vi "LabVIEW Data to Python String (Variant)-[no 2d array support].vi"(8 "error in (no error)":errorcluster, 10 "LabVIEW Data":variant) -> (0 "error out":errorcluster, 2 "Python String":string)   [LabVIEW 2020, in "jki_python_data_tools.lvlib"]
doc: "Writes a value associated with key in a specified section of the configuration data identified by refnum. If \"key\" input is not specified, the name of the variant object is used as the key.\n\nFor example a Boolean named \"Enable\" with a value of TRUE would correspond to the key-value pair:\n\nEnable=TRUE"
uses:
  jki_python_data_tools.lvlib
  LabVIEW Data to Python String/LabVIEW Data to Python String (I64).vi
  LabVIEW Data to Python String/LabVIEW Data to Python String (U64).vi
  LabVIEW Data to Python String/LabVIEW Data to Python String (Boolean).vi
  LabVIEW Data to Python String/LabVIEW Data to Python String (EXT).vi
  LabVIEW Data to Python String/LabVIEW Data to Python String (CXT).vi
  LabVIEW Data to Python String/LabVIEW Data to Python String (Path).vi
  LabVIEW Data to Python String/LabVIEW Data to Python String (String).vi
  LabVIEW Data to Python String/LabVIEW Data to Python String (I32).vi
  LabVIEW Data to Python String/LabVIEW Data to Python String (U32).vi
panel:
  # "Copyright © 2003-2009 JKI. All rights reserved.\n\nAuthor: Jim Kring [jim.kring@jameskring.com]\n\nThis library is provided \"AS IS\" ,WITHOUT WARRANTIES OR \nCONDITIONS OF ANY KIND, either express or implied.\n\nJames Kring, Inc. -- http://www.jameskring.com"
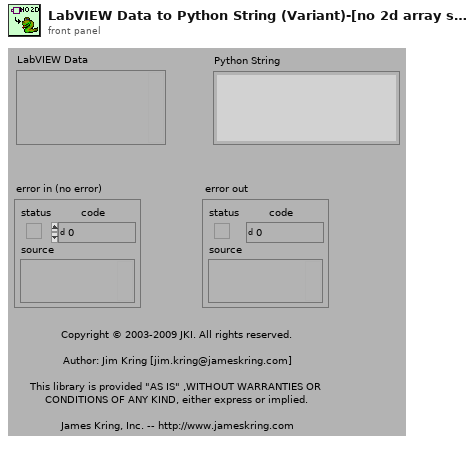
[diagram p1: front panel]
types:
  T1 = typedef "jki_python_data_tools.lvlib/Type Descriptor Enumeration__Py2LV.ctl" = enum8{"<Null>", "I8", "I16", "I32", "I64", "U8", "U16", "U32", "U64", "SGL", "DBL", "EXT", "CSG", "CDB", "CXT", "0x0F", "0x10", "0x11", "0x12", "0x13", "0x14", "Enum U8", "Enum U16", "Enum U32", "Enum U64", "SGL PQ", "DBL PQ", "EXT PQ", "CSG PQ", "CDB PQ", "CXT PQ", "0x1F", "0x20", "Boolean", "0x22", "0x23", "0x24", "0x25", "0x26", "0x27", "0x28", "0x29", "0x2A", "0x2B", "0x2C", "0x2D", "0x2E", "0x2F", "String", "0x31", "Path", "Pict", "0x34", "0x35", "0x36", "DAQ", "0x38", "0x39", "0x3A", "0x3B", "0x3C", "0x3D", "0x3E", "0x3F", "Array", "0x41", "0x42", "0x43", "0x44", "0x45", "0x46", "0x47", "0x48", "0x49", "0x4A", "0x4B", "0x4C", "0x4D", "0x4E", "0x4F", "Cluster", "0x51", "0x52", "Variant", "Waveform", "0x55", "0x56", "0x57", "0x58", "0x59", "0x5A", "0x5B", "0x5C", "0x5D", "0x5E", "0x5F", "0x60", "0x61", "0x62", "0x63", "0x64", "0x65", "0x66", "0x67", "0x68", "0x69", "0x6A", "0x6B", "0x6C", "0x6D", "0x6E", "0x6F", "Refnum"}
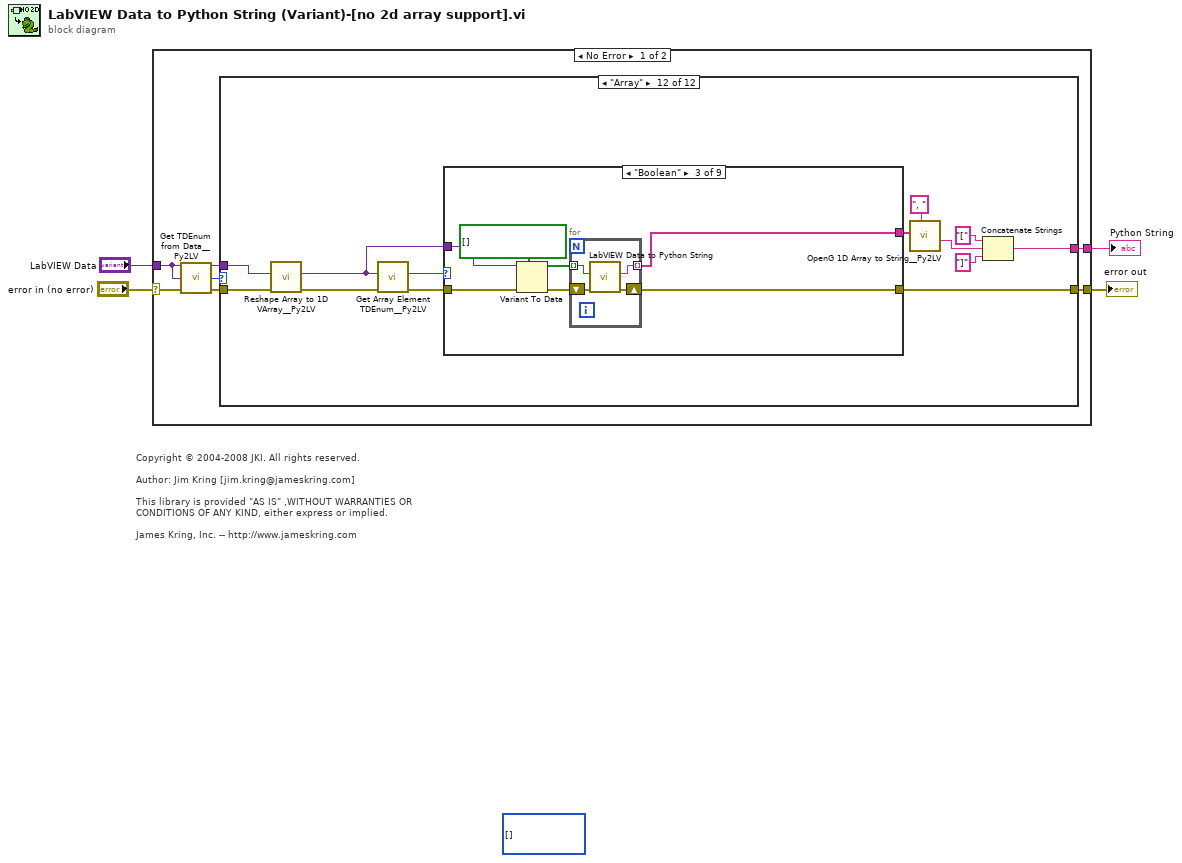
[diagram p0: block diagram]
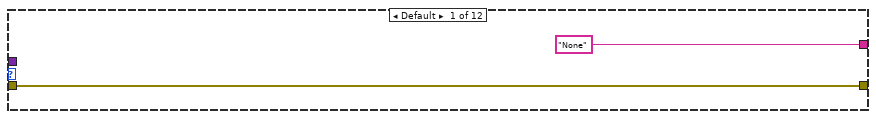
[diagram p2: hidden frame]
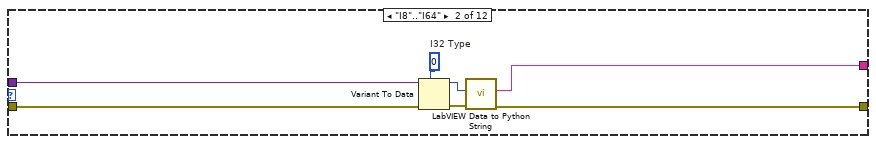
[diagram p3: hidden frame]
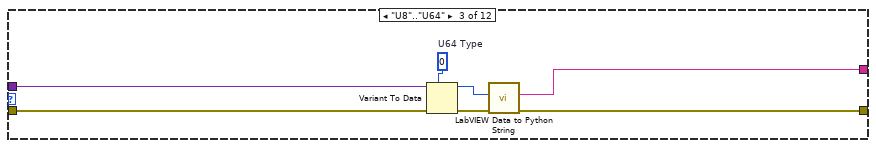
[diagram p4: hidden frame]
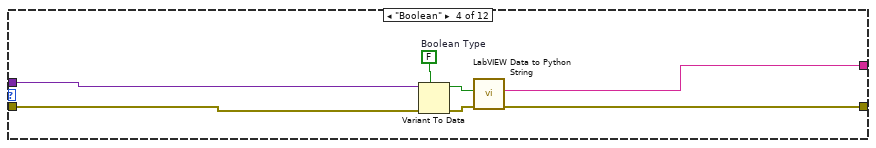
[diagram p5: hidden frame]
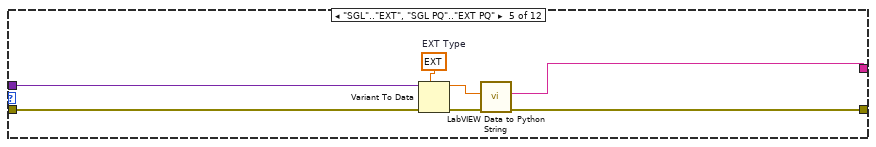
[diagram p6: hidden frame]
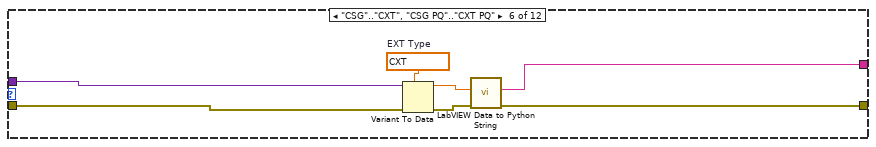
[diagram p7: hidden frame]
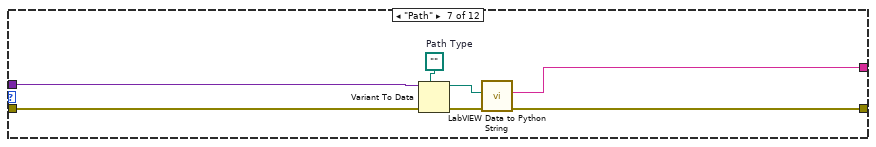
[diagram p8: hidden frame]
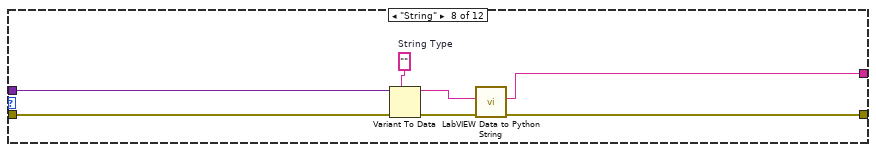
[diagram p9: hidden frame]
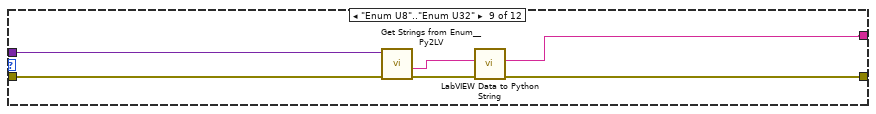
[diagram p10: hidden frame]
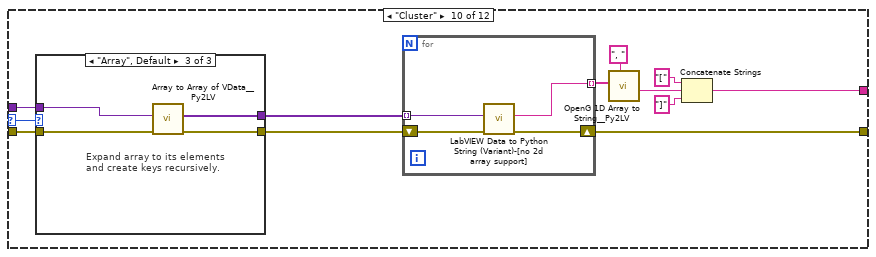
[diagram p11: hidden frame]
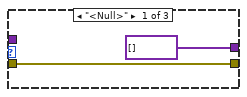
[diagram p12: hidden frame]
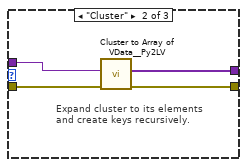
[diagram p13: hidden frame]
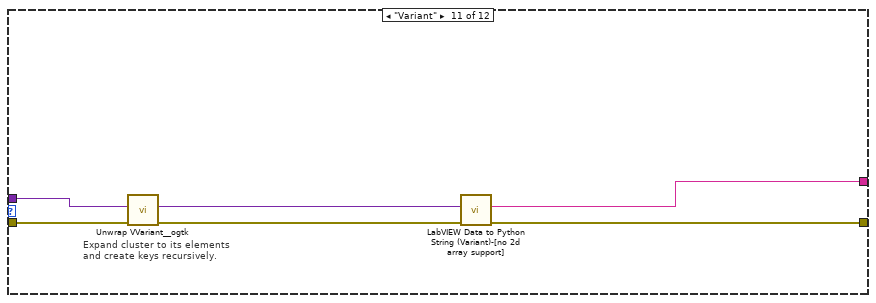
[diagram p14: hidden frame]
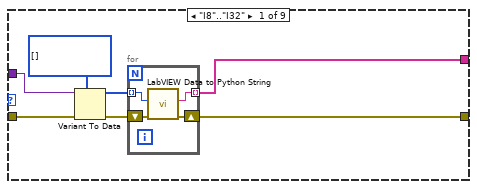
[diagram p15: hidden frame]
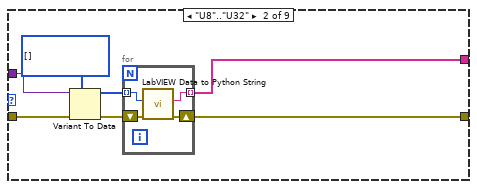
[diagram p16: hidden frame]
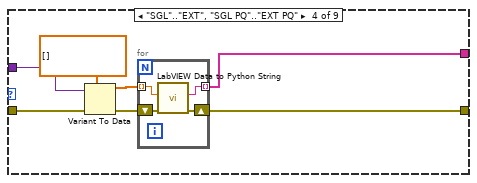
[diagram p17: hidden frame]
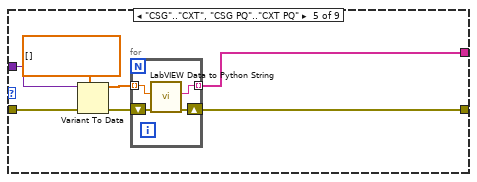
[diagram p18: hidden frame]
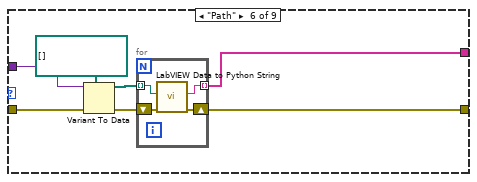
[diagram p19: hidden frame]
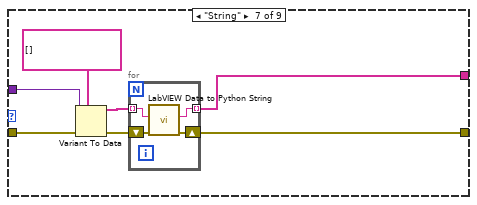
[diagram p20: hidden frame]
diagram:
  (unwired) i32[] []
  # "Copyright © 2004-2008 JKI. All rights reserved.\n\nAuthor: Jim Kring [jim.kring@jameskring.com]\n\nThis library is provided \"AS IS\" ,WITHOUT WARRANTIES OR \nCONDITIONS OF ANY KIND, either express or implied.\n\nJames Kring, Inc. -- http://www.jameskring.com"
  n1 = case shown="No Error" "error in (no error)" {
    selector: "error in (no error)" -> [w8 w204]
    tunnel: [w5 w204] -> w4
    tunnel: "LabVIEW Data" -> [w7 _]
    tunnel: [w6 "None"] -> w1
    frame No Error {
      n2 = call "Get TDEnum from Data__Py2LV.vi"("Data"=w7) -> ("Type Descriptor Enumeration"=w9:T1)  [unwired: 4 in]
      n3 = case shown="\"Array\"" w9 {
        selector: w9 -> [_ _ _ _ _ _ _ _ _ w69 _ _]
        tunnel: w7 -> [_ w17 w24 w31 w38 w46 w52 w59 w65 w78 w98 w100]
        tunnel: w8 -> [w10 w16 w23 w30 w37 w45 w51 w58 w66 w77 w97 w101]
        tunnel: ["None" w12 w20 w26 w33 w40 w48 w55 w61 w70 w95 w104] -> w6
        tunnel: [w10 w13 w19 w27 w34 w42 w47 w54 w62 w68 w94 w103] -> w5
        frame Default {
        }
        frame "I8".."I64" {
          w18 = i64 0  # I32 Type
          n4 = Variant To Data(error in=w16, type=w18, Variant=w17) -> (data=w15:i64, error out=w14:errorcluster)
          n5 = call-poly "LabVIEW Data to Python String.vi"("error in (no error)"=w14, "LabVIEW Data"=w15) -> ("error out"=w13:errorcluster, "Python String"=w12:string)  [unwired: 8 in]
        }
        frame "U8".."U64" {
          w25 = u64 0  # U64 Type
          n6 = Variant To Data(error in=w23, type=w25, Variant=w24) -> (data=w21:u64, error out=w22:errorcluster)
          n7 = call-poly "LabVIEW Data to Python String.vi"("error in (no error)"=w22, "LabVIEW Data"=w21) -> ("error out"=w19:errorcluster, "Python String"=w20:string)  [unwired: 8 in]
        }
        frame "Boolean" {
          w32 = FALSE  # Boolean Type
          n8 = Variant To Data(error in=w30, type=w32, Variant=w31) -> (data=w29:bool, error out=w28:errorcluster)
          n9 = call-poly "LabVIEW Data to Python String.vi"("error in (no error)"=w28, "LabVIEW Data"=w29) -> ("error out"=w27:errorcluster, "Python String"=w26:string)  [unwired: 8 in]
        }
        frame "SGL".."EXT", "SGL PQ".."EXT PQ" {
          w39 = ext 0.0  # EXT Type
          n10 = Variant To Data(error in=w37, type=w39, Variant=w38) -> (data=w36:ext, error out=w35:errorcluster)
          n11 = call-poly "LabVIEW Data to Python String.vi"("error in (no error)"=w35, "LabVIEW Data"=w36) -> ("error out"=w34:errorcluster, "Python String"=w33:string)  [unwired: 8 in]
        }
        frame "CSG".."CXT", "CSG PQ".."CXT PQ" {
          w43 = cxt 0.0+0.0i  # EXT Type
          n12 = Variant To Data(error in=w45, type=w43, Variant=w46) -> (data=w41:cxt, error out=w44:errorcluster)
          n13 = call-poly "LabVIEW Data to Python String.vi"("error in (no error)"=w44, "LabVIEW Data"=w41) -> ("error out"=w42:errorcluster, "Python String"=w40:string)  [unwired: 8 in]
        }
        frame "Path" {
          w53 = path ""  # Path Type
          n14 = Variant To Data(error in=w51, type=w53, Variant=w52) -> (data=w50:path, error out=w49:errorcluster)
          n15 = call-poly "LabVIEW Data to Python String.vi"("error in (no error)"=w49, "LabVIEW Data"=w50) -> ("error out"=w47:errorcluster, "Python String"=w48:string)  [unwired: 8 in]
        }
        frame "String" {
          w60 = ""  # String Type
          n16 = Variant To Data(error in=w58, type=w60, Variant=w59) -> (data=w57:string, error out=w56:errorcluster)
          n17 = call-poly "LabVIEW Data to Python String.vi"("error in (no error)"=w56, "LabVIEW Data"=w57) -> ("error out"=w54:errorcluster, "Python String"=w55:string)  [unwired: 8 in]
        }
        frame "Enum U8".."Enum U32" {
          n18 = call "Get Strings from Enum__Py2LV.vi"("error in (no error)"=w66, "Enum"=w65) -> ("error out"=w63:errorcluster, "String Value"=w64:string)  [unwired: 6 in, 2 out]
          n19 = call-poly "LabVIEW Data to Python String.vi"("error in (no error)"=w63, "LabVIEW Data"=w64) -> ("error out"=w62:errorcluster, "Python String"=w61:string)  [unwired: 8 in]
        }
        frame "Cluster" {
          n20 = case shown="\"Array\", Default" w69 {
            tunnel: w78 -> [_ w84 w86]
            tunnel: w77 -> [w79 w83 w85]
            tunnel: [variant[] [] w81 w88] -> w76
            tunnel: [w79 w82 w87] -> w67
            frame "<Null>" {
            }
            frame "Cluster" {
              # "Expand cluster to its elements\nand create keys recursively."
              n21 = call "Cluster to Array of VData__Py2LV.vi"("error in (no error)"=w83, "Cluster"=w84) -> ("error out"=w82:errorcluster, "Array of VData"=w81:variant[])  [unwired: 8 in]
            }
            frame "Array", Default {
              # "Expand array to its elements\nand create keys recursively."
              n22 = call "Array to Array of VData__Py2LV.vi"("error in (no error)"=w85, "MultiD Array"=w86) -> ("error out"=w87:errorcluster, "1D Array of Variants"=w88:variant[])  [unwired: 8 in]
            }
          }
          n23 = for {
            shift-right: [w90] -> w68
            shift-left: w67 -> [w89]
            tunnel: w76 -> [w92] mode=indexing
            tunnel: [w91] -> w75 mode=indexing
            n24 = call "LabVIEW Data to Python String (Variant)-[no 2d array support].vi"("error in (no error)"=w89, "LabVIEW Data"=w92) -> ("error out"=w90:errorcluster, "Python String"=w91:string)  [unwired: 8 in]
          }
          n25 = call "OpenG 1D Array to String__Py2LV.vi"("delimiter (Tab)"=", ", "Array of Strings"=w75) -> ("delimited string"=w73:string)  [unwired: 9 in]
          n26 = Concatenate Strings("[" ("string"), w73, "]" ("string")) -> (w70:string)
        }
        frame "Variant" {
          # "Expand cluster to its elements\nand create keys recursively."
          n27 = call <userlib>:"Unwrap VVariant__ogtk.vi"("error in (no error)"=w97, "VVariant"=w98) -> ("error out"=w93:errorcluster, "Variant"=w96:variant)  [unwired: 8 in]
          n28 = call "LabVIEW Data to Python String (Variant)-[no 2d array support].vi"("error in (no error)"=w93, "LabVIEW Data"=w96) -> ("error out"=w94:errorcluster, "Python String"=w95:string)  [unwired: 8 in]
        }
        frame "Array" {
          n29 = call "Reshape Array to 1D VArray__Py2LV.vi"("error in (no error)"=w101, "MultiD Array"=w100) -> ("error out"=w102:errorcluster, "1D VArray"=w99:variant)  [unwired: 7 in, 1 out]
          n30 = call "Get Array Element TDEnum__Py2LV.vi"("error in (no error)"=w102, "Array"=w99) -> ("error out"=w107:errorcluster, "Element Type"=w106:T1)  [unwired: 8 in]
          n31 = case shown="\"Boolean\"" w106 {
            tunnel: w99 -> [w118 w123 w137 w147 w157 w169 w180 _ w196]
            tunnel: w107 -> [w112 w124 w136 w148 w156 w170 w181 w192 w197]
            tunnel: [w116 w125 w134 w146 w158 w168 w179 w189 w195] -> w105
            tunnel: [w113 w126 w135 w145 w159 w167 w178 w192 w194] -> w103
            frame "I8".."I32" {
              n32 = Variant To Data(error in=w112, type=i32[] [], Variant=w118) -> (data=w117:i32[], error out=w114:errorcluster)
              n33 = for {
                tunnel: w117 -> [w122] mode=indexing
                tunnel: [w121] -> w116 mode=indexing
                shift-right: [w119] -> w113
                shift-left: w114 -> [w120]
                n34 = call-poly "LabVIEW Data to Python String.vi"("error in (no error)"=w120, "LabVIEW Data"=w122) -> ("error out"=w119:errorcluster, "Python String"=w121:string)  [unwired: 8 in]
              }
            }
            frame "U8".."U32" {
              n35 = Variant To Data(error in=w124, type=u32[] [], Variant=w123) -> (data=w129:u32[], error out=w127:errorcluster)
              n36 = for {
                tunnel: w129 -> [w133] mode=indexing
                tunnel: [w132] -> w125 mode=indexing
                shift-right: [w130] -> w126
                shift-left: w127 -> [w131]
                n37 = call-poly "LabVIEW Data to Python String.vi"("error in (no error)"=w131, "LabVIEW Data"=w133) -> ("error out"=w130:errorcluster, "Python String"=w132:string)  [unwired: 8 in]
              }
            }
            frame "Boolean" {
              n38 = Variant To Data(error in=w136, type=bool[] [], Variant=w137) -> (data=w140:bool[], error out=w138:errorcluster)
              n39 = for {
                tunnel: w140 -> [w144] mode=indexing
                tunnel: [w143] -> w134 mode=indexing
                shift-right: [w141] -> w135
                shift-left: w138 -> [w142]
                n40 = call-poly "LabVIEW Data to Python String.vi"("error in (no error)"=w142, "LabVIEW Data"=w144) -> ("error out"=w141:errorcluster, "Python String"=w143:string)  [unwired: 8 in]
              }
            }
            frame "SGL".."EXT", "SGL PQ".."EXT PQ" {
              n41 = Variant To Data(error in=w148, type=ext[] [], Variant=w147) -> (data=w151:ext[], error out=w149:errorcluster)
              n42 = for {
                tunnel: w151 -> [w155] mode=indexing
                tunnel: [w154] -> w146 mode=indexing
                shift-right: [w152] -> w145
                shift-left: w149 -> [w153]
                n43 = call-poly "LabVIEW Data to Python String.vi"("error in (no error)"=w153, "LabVIEW Data"=w155) -> ("error out"=w152:errorcluster, "Python String"=w154:string)  [unwired: 8 in]
              }
            }
            frame "CSG".."CXT", "CSG PQ".."CXT PQ" {
              n44 = Variant To Data(error in=w156, type=cxt[] [], Variant=w157) -> (data=w162:cxt[], error out=w160:errorcluster)
              n45 = for {
                tunnel: w162 -> [w166] mode=indexing
                tunnel: [w165] -> w158 mode=indexing
                shift-right: [w163] -> w159
                shift-left: w160 -> [w164]
                n46 = call-poly "LabVIEW Data to Python String.vi"("error in (no error)"=w164, "LabVIEW Data"=w166) -> ("error out"=w163:errorcluster, "Python String"=w165:string)  [unwired: 8 in]
              }
            }
            frame "Path" {
              n47 = Variant To Data(error in=w170, type=path[] [], Variant=w169) -> (data=w173:path[], error out=w171:errorcluster)
              n48 = for {
                tunnel: w173 -> [w177] mode=indexing
                tunnel: [w176] -> w168 mode=indexing
                shift-right: [w174] -> w167
                shift-left: w171 -> [w175]
                n49 = call-poly "LabVIEW Data to Python String.vi"("error in (no error)"=w175, "LabVIEW Data"=w177) -> ("error out"=w174:errorcluster, "Python String"=w176:string)  [unwired: 8 in]
              }
            }
            frame "String" {
              n50 = Variant To Data(error in=w181, type=string[] [], Variant=w180) -> (data=w184:string[], error out=w182:errorcluster)
              n51 = for {
                tunnel: w184 -> [w188] mode=indexing
                tunnel: [w187] -> w179 mode=indexing
                shift-right: [w185] -> w178
                shift-left: w182 -> [w186]
                n52 = call-poly "LabVIEW Data to Python String.vi"("error in (no error)"=w186, "LabVIEW Data"=w188) -> ("error out"=w185:errorcluster, "Python String"=w187:string)  [unwired: 8 in]
              }
            }
            frame Default {
              n53 = Initialize Array("", 0 ("dimension size")) -> (w189:string[])
            }
            frame "Enum U8".."Enum U32", "Cluster" {
              n54 = call "Array to Array of VData__Py2LV.vi"("error in (no error)"=w197, "MultiD Array"=w196) -> ("error out"=w193:errorcluster, "1D Array of Variants"=w198:variant[])  [unwired: 8 in]
              n55 = for {
                shift-right: [w200] -> w194
                shift-left: w193 -> [w201]
                tunnel: w198 -> [w202] mode=indexing
                tunnel: [w199] -> w195 mode=indexing
                n56 = call "LabVIEW Data to Python String (Variant)-[no 2d array support].vi"("error in (no error)"=w201, "LabVIEW Data"=w202) -> ("error out"=w200:errorcluster, "Python String"=w199:string)  [unwired: 8 in]
              }
            }
          }
          n57 = call "OpenG 1D Array to String__Py2LV.vi"("delimiter (Tab)"=", ", "Array of Strings"=w105) -> ("delimited string"=w110:string)  [unwired: 9 in]
          n58 = Concatenate Strings("[" ("string"), w110, "]" ("string")) -> (w104:string)
        }
      }
    }
    frame Error {
    }
  }
  "error out" <- w4
  "Python String" <- w1
